vi "motortestMeng4XY3.vi"() -> ()   [LabVIEW 2014]
doc: "Shows how to perform a relative motor move."
uses:
  <vilib>/Utility/inputDevices.llb/joystickAcquire.vi
  <vilib>/Utility/inputDevices.llb/closeJoystick.vi
panel:
  out "Position Z":sgl=0.29786614
  out "Position X":sgl=-2.4631822
  in  "Stop":bool
  in  "MG17Motor Z":refnum<k7>(container)
  in  "Motor settings (Z)":cluster{"Vmax (mm/s)":sgl, "Acc (mm/s/s)":sgl}={"Vmax (mm/s)"=0.03, "Acc (mm/s/s)"=1.0}
  out "Position Y":sgl=-1.2969333
  in  "Motor settings (X,Y)":cluster{"Vmax (mm/s)":sgl, "Acc (mm/s/s)":sgl}={"Vmax (mm/s)"=0.05, "Acc (mm/s/s)"=0.5}
  in  "Motor Limits":T1={"XMAX"=8.5, "XMIN"=-5.0, "YMAX"=6.0, "YMIN"=-6.0, "ZMAX"=0.33, "ZMIN"=0.25}
  in  "MG17Motor Y":refnum<k7>(container)
  out "axis info":T2={"X axis"=-256, "Y axis"=-256, "Z axis"=-32768, "X axis rotation"=0, "Y axis rotation"=0, "Z axis rotation"=0, "U axis"=0, "V axis"=0}
  out "button info":T3
  in  "MG17Motor X":refnum<k7>(container)
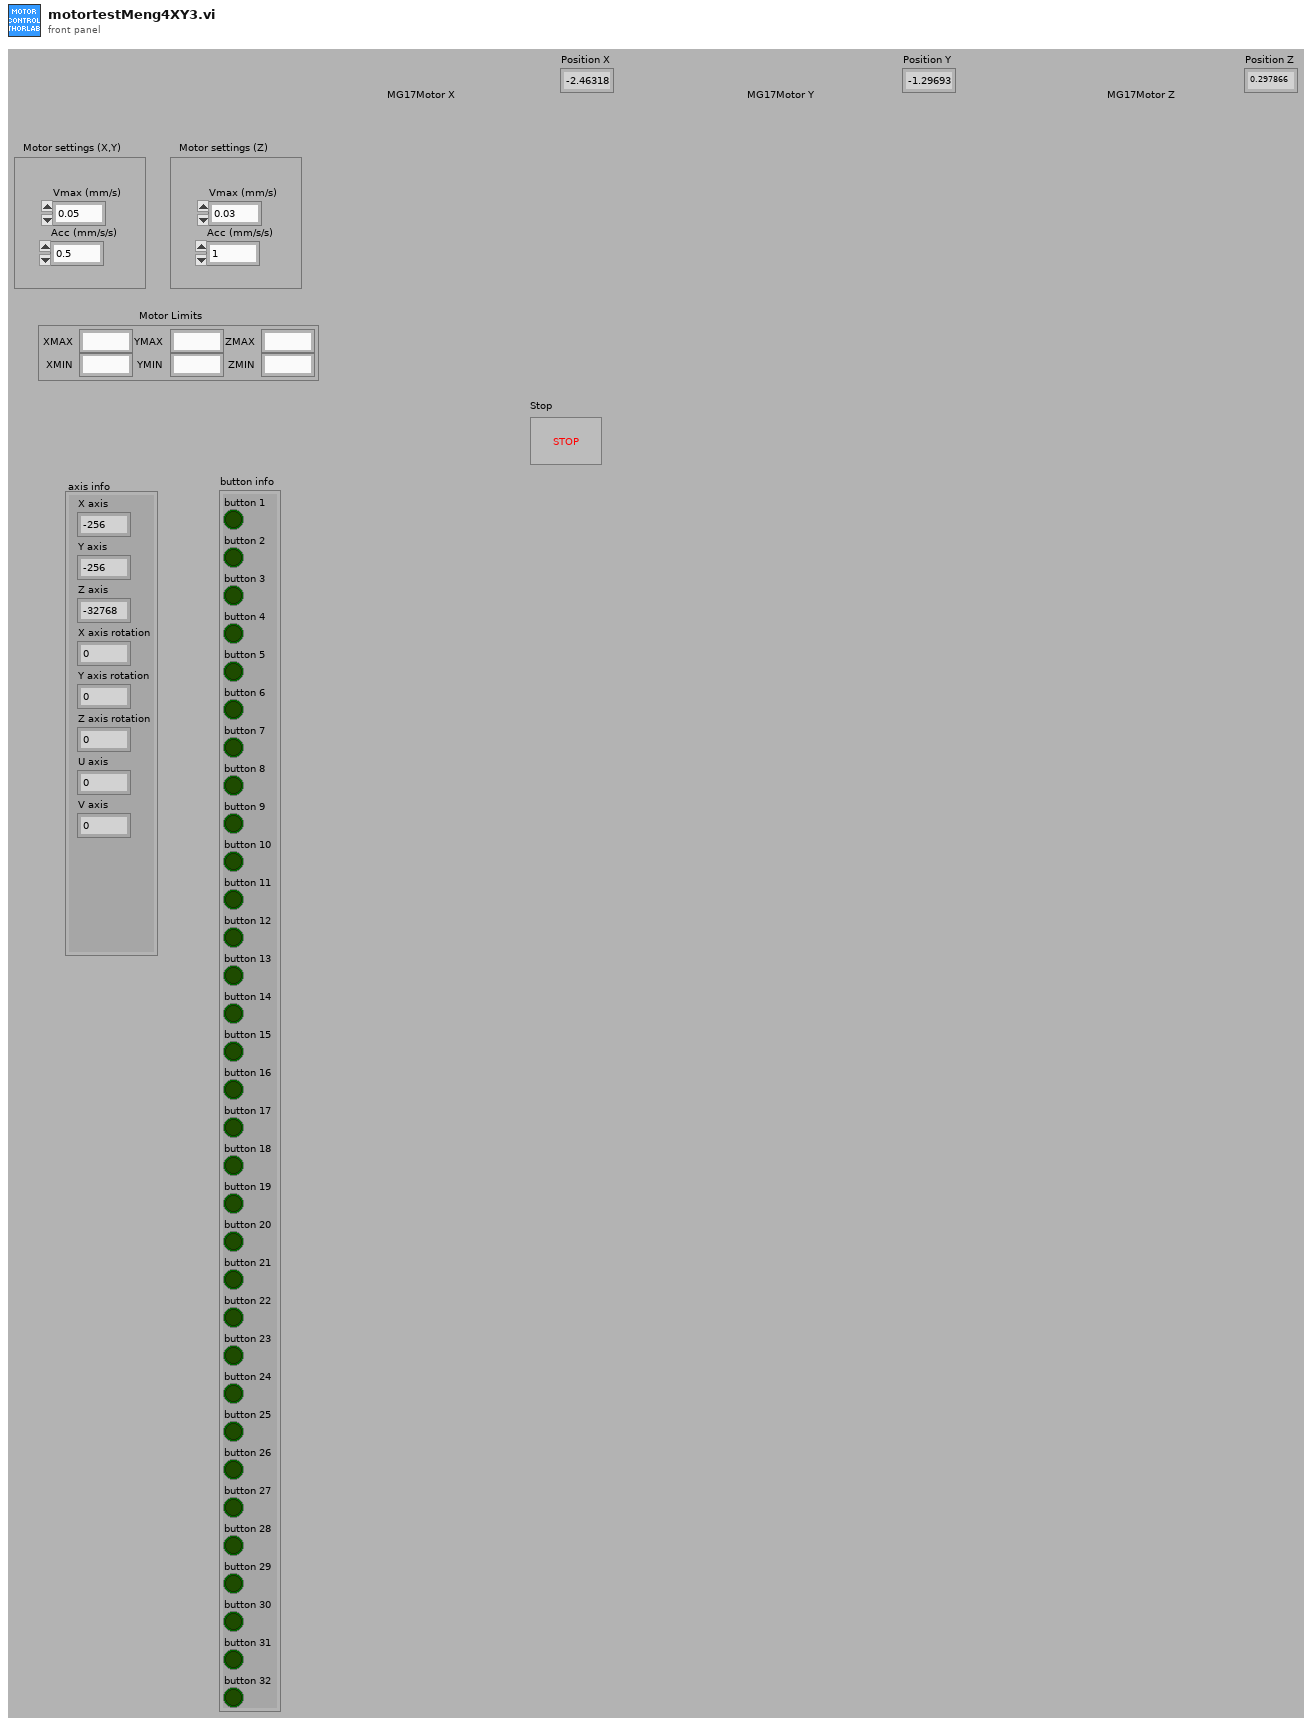
[diagram p1: front panel]
types:
  T1 = cluster{"XMAX":sgl, "XMIN":sgl, "YMAX":sgl, "YMIN":sgl, "ZMAX":sgl, "ZMIN":sgl}
  T2 = cluster{"X axis":i32, "Y axis":i32, "Z axis":i32, "X axis rotation":i32, "Y axis rotation":i32, "Z axis rotation":i32, "U axis":i32, "V axis":i32}
  T3 = cluster{"button 1":bool, "button 2":bool, "button 3":bool, "button 4":bool, "button 5":bool, "button 6":bool, "button 7":bool, "button 8":bool, "button 9":bool, "button 10":bool, "button 11":bool, "button 12":bool, "button 13":bool, "button 14":bool, "button 15":bool, "button 16":bool, "button 17":bool, "button 18":bool, "button 19":bool, "button 20":bool, "button 21":bool, "button 22":bool, "button 23":bool, "button 24":bool, "button 25":bool, "button 26":bool, "button 27":bool, "button 28":bool, "button 29":bool, "button 30":bool, "button 31":bool, "button 32":bool}
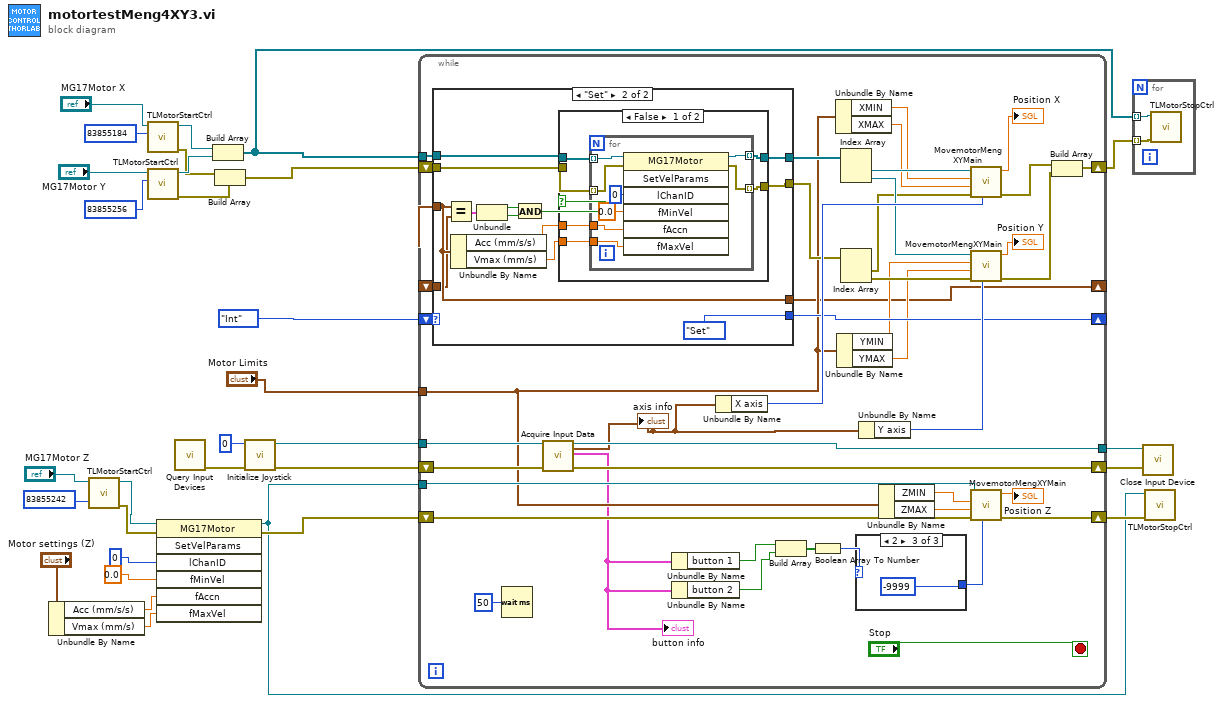
[diagram p0: block diagram]
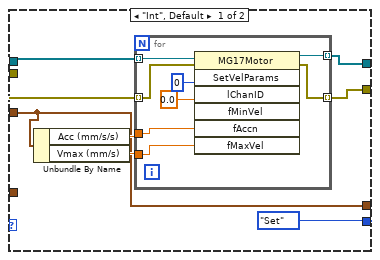
[diagram p2: hidden frame]
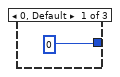
[diagram p4: hidden frame]
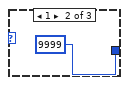
[diagram p5: hidden frame]
diagram:
  n1 = Unbundle By Name("Motor settings (Z)") -> ("Acc (mm/s/s)"=w19:sgl, "Vmax (mm/s)"=w20:sgl)
  n2 = call "TLMotorStartCtrl.vi"("SerialNum"=83855242 ("lChanID"), "Motor Ref"="MG17Motor Z") -> ("Error Out"=w18:errorcluster, "Motor Ref"=w17:refnum<k7>)  [unwired: 4 in]
  n3 = call "TLMotorStartCtrl.vi"("SerialNum"=83855184 ("lChanID"), "Motor Ref"="MG17Motor X") -> ("Error Out"=w7:errorcluster, "Motor Ref"=w8:refnum<k7>)  [unwired: 4 in]
  n4 = call "TLMotorStartCtrl.vi"("SerialNum"=83855256 ("lChanID"), "Motor Ref"="MG17Motor Y") -> ("Error Out"=w6:errorcluster, "Motor Ref"=w9:refnum<k7>)  [unwired: 4 in]
  n5 = invoke class="MG17Motor" method="SetVelParams"(reference=w17, error in=w18, "lChanID"=0, "fMinVel"=sgl 0.0, "fAccn"=w19, "fMaxVel"=w20) -> (reference out=w11:refnum<k7>, error out=w13:errorcluster)  [unwired: 1 in, 5 out]
  n6 = call <vilib>:"Query Input Devices.vi"() -> ("error out"=w30:errorcluster)  [unwired: 8 in, 3 out]
  n7 = Build Array(w8, w9) -> (w4:refnum<k7>[])
  n8 = Build Array(w7, w6) -> (w5:errorcluster[])
  n9 = call <vilib>:"Initialize Joystick.vi"("error in (no error)"=w30, "device index"=0) -> ("error out"=w1:errorcluster, "device ID"=w29:refnum<k1>)  [unwired: 8 in]
  n10 = while {
    tunnel: w29 -> [w75]
    tunnel: [w74] -> w28
    tunnel: w11 -> [w61]
    shift-right: [w62] -> w12
    shift-left: w13 -> [w60]
    shift-right: [w56] -> _
    shift-left: enum16{"Int", "Set"}."Int" ("Enum") -> [w57]
    shift-right: [w35] -> _
    shift-left: _ -> [w34]
    tunnel: w4 -> [w49]
    shift-right: [w45] -> w3
    shift-left: w5 -> [w48]
    tunnel: "Motor Limits" -> [w39]
    shift-right: [w73] -> w27
    shift-left: w1 -> [w40]
    stop <- "Stop" stop-if-true
    n11 = case shown="\"Set\"" w57 {
      tunnel: [w78 w97] -> w55
      tunnel: [w77 w103] -> w52
      tunnel: w48 -> [w83 w104]
      tunnel: [enum16{"Int", "Set"}."Set" ("Enum") enum16{"Int", "Set"}."Set" ("Enum")] -> w56
      tunnel: w49 -> [w79 w98]
      tunnel: "Motor settings (X,Y)" -> [w76 w96]
      tunnel: [w76 w96] -> w35
      tunnel: w34 -> [_ w92]
      frame "Int", Default {
        n12 = Unbundle By Name(w76) -> ("Acc (mm/s/s)"=w82:sgl, "Vmax (mm/s)"=w81:sgl)
        n13 = for {
          tunnel: w82 -> [w85]
          tunnel: w81 -> [w84]
          tunnel: w79 -> [w91] mode=indexing
          tunnel: [w88] -> w78 mode=indexing
          tunnel: w83 -> [w87] mode=indexing
          tunnel: [w86] -> w77 mode=indexing
          n14 = invoke class="MG17Motor" method="SetVelParams"(reference=w91, error in=w87, "lChanID"=0, "fMinVel"=sgl 0.0, "fAccn"=w85, "fMaxVel"=w84) -> (reference out=w88:refnum<k7>, error out=w86:errorcluster)  [unwired: 1 in, 5 out]
        }
      }
      frame "Set" {
        n15 = Equal?(x=w96, y=w92) -> (x = y?=w94:cluster{"Vmax (mm/s)":bool, "Acc (mm/s/s)":bool})
        n16 = Unbundle By Name(w96) -> ("Acc (mm/s/s)"=w102:sgl, "Vmax (mm/s)"=w101:sgl)
        n17 = Unbundle(w94) -> ("Vmax (mm/s)"=w95:bool, "Acc (mm/s/s)"=w93:bool)
        n18 = And(x=w95, y=w93) -> (x .and. y?=w99:bool)
        n19 = case shown="False" w99 {
          tunnel: w104 -> [w110 w120]
          tunnel: w98 -> [w109 w119]
          tunnel: [w105 w120] -> w103
          tunnel: [w106 w119] -> w97
          tunnel: w102 -> [w108 _]
          tunnel: w101 -> [w107 _]
          frame False {
            n20 = for {
              tunnel: w108 -> [w112]
              tunnel: w107 -> [w111]
              tunnel: w109 -> [w117] mode=indexing
              tunnel: w110 -> [w118] mode=indexing
              tunnel: [w114] -> w106 mode=indexing
              tunnel: [w113] -> w105 mode=indexing
              n21 = invoke class="MG17Motor" method="SetVelParams"(reference=w117, error in=w118, "lChanID"=0, "fMinVel"=sgl 0.0, "fAccn"=w112, "fMaxVel"=w111) -> (reference out=w114:refnum<k7>, error out=w113:errorcluster)  [unwired: 1 in, 5 out]
            }
          }
          frame True {
          }
        }
      }
    }
    n22 = Wait (ms)(milliseconds to wait=u32 50) -> ()  [unwired: 1 out]
    n23 = call-poly <vilib>:"Acquire Input Data.vi"("device ID"=w75, "error in (no error)"=w40) -> ("device ID"=w74:refnum<k1>, "axis info"=w71:T2, "button info"=w33:T3, "error out"=w73:errorcluster)  [unwired: 13 in, 1 out]
    "axis info" <- w71
    "button info" <- w33
    n24 = Unbundle By Name(w33) -> ("button 1"=w66:bool)
    n25 = Unbundle By Name(w33) -> ("button 2"=w65:bool)
    n26 = Unbundle By Name(w71) -> ("X axis"=w69:i32)
    n27 = Build Array(w66, w65) -> (w64:bool[])
    n28 = Boolean Array To Number(Boolean array=w64) -> (number=w59:u32)
    n29 = Unbundle By Name(w39) -> ("XMIN"=w44:sgl, "XMAX"=w43:sgl)
    n30 = Unbundle By Name(w39) -> ("YMIN"=w42:sgl, "YMAX"=w41:sgl)
    n31 = Index Array(array=w55) -> (element #1=w54:refnum<k7>, element #2=w53:refnum<k7>)  [unwired: 2 in]
    n32 = Index Array(array=w52) -> (element #1=w51:errorcluster, element #2=w50:errorcluster)  [unwired: 2 in]
    n33 = case shown="2" w59 {
      tunnel: [0 ("Y axis") 9999 ("Y axis") -9999 ("Y axis")] -> w58
      frame 0, Default {
      }
      frame 1 {
      }
      frame 2 {
      }
    }
    n34 = Unbundle By Name(w71) -> ("Y axis"=w67:i32)
    n35 = Unbundle By Name(w39) -> ("ZMIN"=w38:sgl, "ZMAX"=w37:sgl)
    n36 = call "MovemotorMengXYMain.vi"("Joystick axis"=w69, "error in (no error)"=w51, "XorYMAX"=w43, "XorYMIN"=w44, "Automation Refnum in"=w54) -> ("error out"=w47:errorcluster, "XorYPosition"=→"Position X":sgl)  [unwired: 4 in, 1 out]
    n37 = call "MovemotorMengXYMain.vi"("Joystick axis"=w67, "error in (no error)"=w50, "XorYMAX"=w41, "XorYMIN"=w42, "Automation Refnum in"=w53) -> ("error out"=w46:errorcluster, "XorYPosition"=→"Position Y":sgl)  [unwired: 4 in, 1 out]
    n38 = call "MovemotorMengXYMain.vi"("Joystick axis"=w58, "error in (no error)"=w60, "XorYMAX"=w37, "XorYMIN"=w38, "Automation Refnum in"=w61) -> ("error out"=w62:errorcluster, "XorYPosition"=→"Position Z":sgl)  [unwired: 4 in, 1 out]
    n39 = Build Array(w47, w46) -> (w45:errorcluster[])
  }
  n40 = for {
    tunnel: w4 -> [w125] mode=indexing
    tunnel: w3 -> [w124] mode=indexing
    n41 = call "TLMotorStopCtrl.vi"("Error In (No Error)"=w124, "Motor Ref"=w125) -> ()  [unwired: 4 in, 2 out]
  }
  n42 = call-poly <vilib>:"Close Input Device.vi"("error in (no error)"=w27, "device ID"=w28) -> ()  [unwired: 8 in, 1 out]
  n43 = call "TLMotorStopCtrl.vi"("Error In (No Error)"=w12, "Motor Ref"=w11) -> ()  [unwired: 4 in, 2 out]
